vi "Not A Session - valid session - returns false.vi"() -> ()   [LabVIEW 2017, in "unit_tests.lvlib"]
uses:
  unit_tests.lvlib
  libssh2/libssh2_init_default.vi
  libssh2/libssh2_session_init_ex.vi
  libssh2/libssh2.lvlib
  <vilib>/PNR/Transparent Assertions/Transparent Assertions/Transparent Assertions.lvlib
panel:
  out "error out":errorcluster
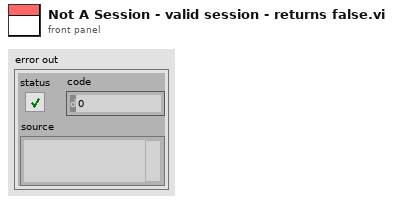
[diagram p1: front panel]
types:
  T1 = typedef "libssh2.lvlib/Session Refnum.ctl" = refnum<k1>
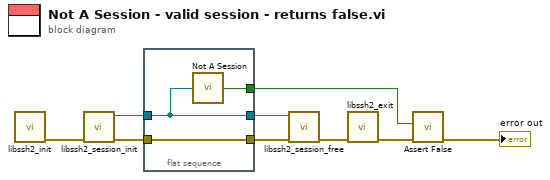
[diagram p0: block diagram]
diagram:
  n1 = call-poly "libssh2_init.vi"() -> ("error out"=w9:errorcluster)  [unwired: 11 in]
  n2 = call "libssh2_session_init.vi"("error in (no error)"=w9) -> ("error out"=w2:errorcluster, "session"=w4:T1)  [unwired: 9 in]
  n3 = flat-sequence {
    tunnel: [w12] -> w5
    tunnel: w4 -> [w10]
    tunnel: [w11] -> w3
    tunnel: w2 -> [w11]
    tunnel: [w10] -> w1
    frame #0 {
      n4 = call "Not A Session.vi"("session"=w10) -> ("Not a Session?"=w12:bool)
    }
  }
  n5 = call "libssh2_session_free.vi"("error in (no error)"=w3, "session"=w1) -> ("error out"=w7:errorcluster)  [unwired: 9 in]
  n6 = call "libssh2_exit.vi"("error in (no error)"=w7) -> ("error out"=w6:errorcluster)  [unwired: 10 in]
  n7 = call <vilib>:"Assert False.vi"("error in (no error)"=w6, "Condition"=w5) -> ("error out"=→"error out":errorcluster)  [unwired: 9 in]
